vi "Vertical Cull and Group.vi"(6 "Line Border":cluster{"Top":dbl, "Bottom":dbl}={"Top"=6.0, "Bottom"=1.0}, 9 "Score Cutoff":dbl=3.0, 10 "Sorted Data":dbl[][](array[numeric])) -> (0 "Rect":T1, 1 "Line":T1, 2 "Score":dbl, 3 "Center":cluster{"X":dbl, "Y":dbl})   [LabVIEW 2016]
doc: "Examine the particle measurements to find the most likely pair that make up the target. This mostly compares the edges of the bounding boxes. It then returns information about the overall target, notably the rectangle sourrounding the particles, the vertical line that bisects the target, and the center of the top particle."
panel:
  out "Grouping Scores":T2(array[cluster])
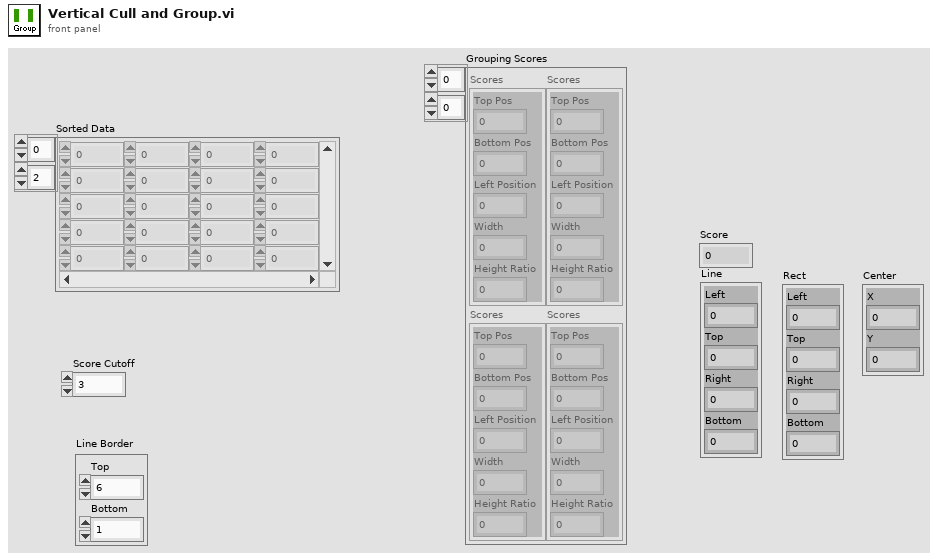
[diagram p1: front panel]
types:
  T1 = cluster{"Left":dbl, "Top":dbl, "Right":dbl, "Bottom":dbl}
  T2 = cluster{"Top Pos":dbl, "Bottom Pos":dbl, "Left Position":dbl, "Width":dbl, "Height Ratio":dbl}[][]
  T3 = cluster{"Top Position":dbl, "Bottom Position":dbl, "Left Gap":dbl, "Width":dbl, "Height Ratio":dbl}
  T4 = cluster{"Left":dbl, "Numeric":dbl, "Right":dbl, "Numeric":dbl}
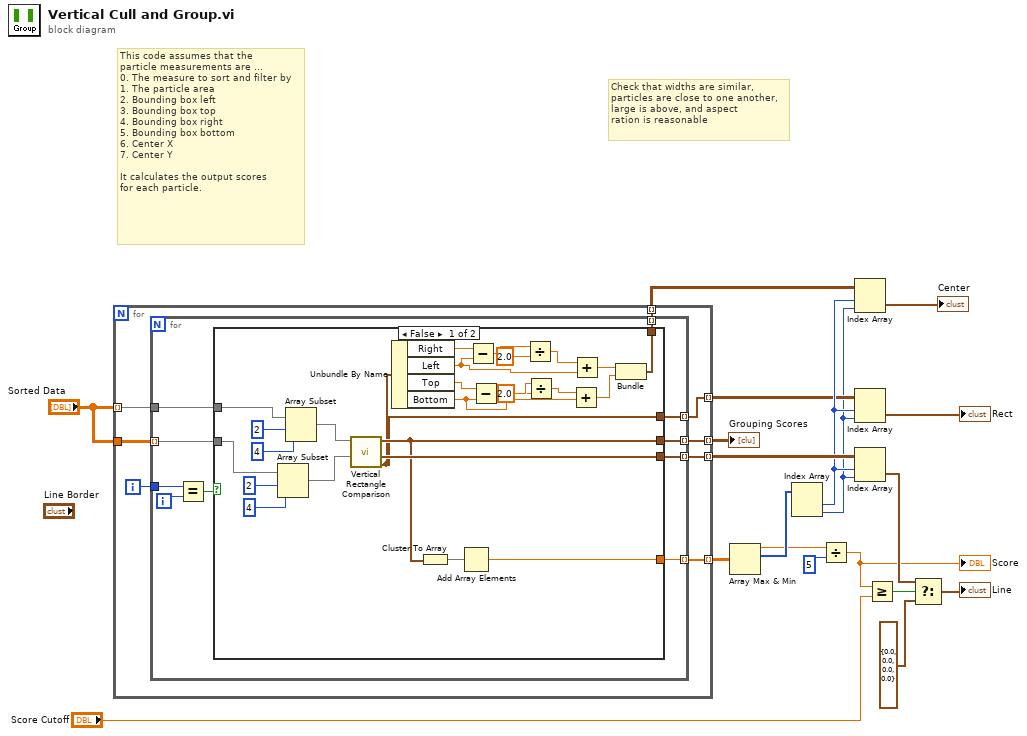
[diagram p0: block diagram]
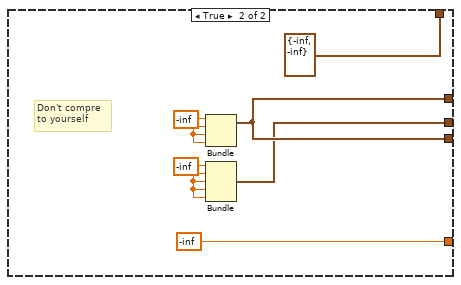
[diagram p2: hidden frame]
diagram:
  # "Check that widths are similar,\nparticles are close to one another,\nlarge is above, and aspect\nration is reasonable"
  # "This code assumes that the\nparticle measurements are ...\n0. The measure to sort and filter by\n1. The particle area\n2. Bounding box left\n3. Bounding box top\n4. Bounding box right\n5. Bounding box bottom\n6. Center X\n7. Center Y\n\nIt calculates the output scores\nfor each particle."
  n1 = for {
    tunnel: "Sorted Data" -> [w27] mode=indexing
    tunnel: "Sorted Data" -> [w26]
    tunnel: [w25] -> w19 mode=indexing
    tunnel: [w23] -> w18 mode=indexing
    tunnel: [w22] -> w15 mode=indexing
    tunnel: [w21] -> w4 mode=indexing
    tunnel: [w20] -> w3 mode=indexing
    i -> [w24]
    n2 = for {
      tunnel: w27 -> [w37]
      tunnel: w26 -> [w35] mode=indexing
      tunnel: [w34] -> w25 mode=indexing
      tunnel: w24 -> [w33]
      tunnel: [w31] -> w23 mode=indexing
      tunnel: [w30] -> w22 mode=indexing
      tunnel: [w29] -> w21 mode=indexing
      tunnel: [w28] -> w20 mode=indexing
      i -> [w32]
      n3 = Equal?(x=w33, y=w32) -> (x = y?=w36:bool)
      n4 = case shown="False" w36 {
        tunnel: w37 -> [w61 _]
        tunnel: w35 -> [w58 _]
        tunnel: [w52 w65] -> w34
        tunnel: [w56 -inf] -> w31
        tunnel: [w53 w68] -> w30
        tunnel: [w51 w68] -> w29
        tunnel: [w50 cluster{dbl, dbl} {-inf, -inf}] -> w28
        frame False {
          n5 = Array Subset(array=w58, index=2, length=4) -> (w54:dbl[])
          n6 = Array Subset(array=w61, index=2, length=4) -> (w55:dbl[])
          n7 = call "Vertical Rectangle Comparison.vi"("Second"=w54, "First"=w55) -> ("Rect"=w51:T1, "Line"=w53:T1, "Scores"=w52:T3)  [unwired: 7 in]
          n8 = Unbundle By Name(w51) -> ("Right"=w49:dbl, "Left"=w46:dbl, "Top"=w48:dbl, "Bottom"=w47:dbl)
          n9 = Cluster To Array(cluster=w52) -> (array=w57:dbl[])
          n10 = Add Array Elements(numeric array=w57) -> (sum=w56:dbl)
          n11 = Subtract(x=w49, y=w46) -> (x-y=w43:dbl)
          n12 = Subtract(x=w48, y=w47) -> (x-y=w39:dbl)
          n13 = Divide(x=w43, y=2.0) -> (x/y=w41:dbl)
          n14 = Divide(x=w39, y=2.0) -> (x/y=w40:dbl)
          n15 = Add(x=w40, y=w47) -> (x+y=w44:dbl)
          n16 = Add(x=w41, y=w46) -> (x+y=w45:dbl)
          n17 = Bundle(w45, w44) -> (w50:cluster{dbl, dbl})  [unwired: 1 in]
        }
        frame True {
          w66 = -inf
          w67 = -inf
          # "Don't compre\nto yourself"
          n18 = Bundle(w67, w67, w67, w67) -> (w68:cluster{dbl, dbl, dbl, dbl})  [unwired: 1 in]
          n19 = Bundle(w66, w66, w66, w66, w66) -> (w65:cluster{dbl, dbl, dbl, dbl, dbl})  [unwired: 1 in]
        }
      }
    }
  }
  "Grouping Scores" <- w19
  n20 = Array Max & Min(array=w18) -> (max value=w7:dbl, max index (indices)=w8:i32[])  [unwired: 2 out]
  n21 = Index Array(array=w8) -> (element #1=w9:i32, element #2=w1:i32)  [unwired: 2 in]
  n22 = Divide(x=w7, y=5 ("length")) -> (x/y=w6:dbl)
  "Score" <- w6
  n23 = Index Array(array=w3, index (row)=w9, index (col)=w1) -> (element=→"Center":cluster{dbl, dbl})
  n24 = Index Array(array=w4, index (row)=w9, index (col)=w1) -> (element=→"Rect":T1)
  n25 = Index Array(array=w15, index (row)=w9, index (col)=w1) -> (element=w14:T1)
  n26 = Greater Or Equal?(x=w6, y="Score Cutoff") -> (x >= y?=w17:bool)
  n27 = Select(t=w14, s=w17, f=cluster{dbl, "Numeric":dbl, dbl, "Numeric":dbl} {0.0, "Numeric"=0.0, 0.0, "Numeric"=0.0}) -> (s? t:f=→"Line":T4)
